vi "Msg Execute.vi"(10 "Msg":refnum<class "Msg.lvclass">, 11 "TEMPLATE Actor in":refnum<class "TEMPLATE Actor.lvclass">) -> (3 "TEMPLATE Actor out":refnum<class "TEMPLATE Actor.lvclass">)   [LabVIEW 2020, in "_Template.lvlib" / "Templates.lvlib" / "TEMPLATE Actor.lvlib" / "TEMPLATE Actor.lvclass"]
uses:
  TEMPLATE Actor.lvclass
  C:/git/jettl/src/jettl/jettl/Actor/Actor/Actor.lvclass
  jettl/jettl/Msg/Msg.lvclass
  TEMPLATE Actor.lvclass/TEMPLATE Actor.ctl
  jettl/jettl/Actor/Actor/Actor.lvclass
  jettl/jettl/Actor/Actor.lvlib
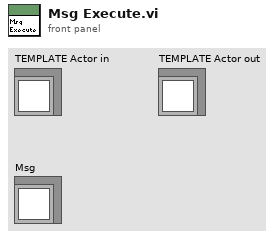
[diagram p1: front panel]
types:
  T1 = typedef "jettl.lvlib/Actor.lvlib/Msgs.ctl" = set{refnum<class "Msg.lvclass">}
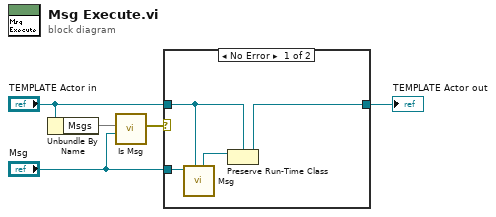
[diagram p0: block diagram]
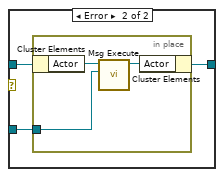
[diagram p2: hidden frame]
diagram:
  n1 = Unbundle By Name("TEMPLATE Actor in") -> ("Msgs"=w5:T1)
  n2 = call "Is Msg.vi"("Msg"="Msg", "Msgs"=w5) -> ("Error"=w4:errorcluster)  [unwired: 9 in]
  n3 = case shown="No Error" w4 {
    tunnel: "TEMPLATE Actor in" -> [w7 w12]
    tunnel: [w6 w11] -> w2
    tunnel: "Msg" -> [w9 w10]
    frame No Error {
      n4 = call-dynamic "Msg.vi"("Actor in"=w7, "Msg in"=w9) -> ("Actor out"=w8:refnum<class "Actor.lvclass">)  [unwired: 9 in]
      n5 = Preserve Run-Time Class(object in=w8, 2:w7) -> (object out=w6:refnum<class "TEMPLATE Actor.lvclass">)  [unwired: 1 in, 1 out]
    }
    frame Error {
      n6 = in-place {
        in-place-border: w10 -> [w13]
        n7 = in-place-cluster #1(w12) -> ("Actor"=w15:refnum<class "Actor.lvclass">)
        n8 = call-dynamic "Msg Execute.vi"("Msg"=w13, "Actor in"=w15) -> ("Actor out"=w14:refnum<class "Actor.lvclass">)  [unwired: 9 in]
        n9 = in-place-cluster #1("Actor"=w14) -> (w11:refnum<class "TEMPLATE Actor.lvclass">)
      }
    }
  }
  "TEMPLATE Actor out" <- w2
